vi "Read.vi"(6 "Append Index":i32, 8 "error in (no error)":errorcluster, 11 "DAT in":refnum<class "LV-Data.DAT.lvclass">) -> (0 "error out":errorcluster, 1 "Notes":string, 2 "Data (Dictionary)":T1[](array[typedef]), 3 "DAT out":refnum<class "LV-Data.DAT.lvclass">, 5 "Path out":path)   [LabVIEW 2016, in "LV-Data.DAT.lvclass"]
uses:
  LV-Data.DAT.lvclass
  C:/Users/patrick/Documents/GitHub/LV-to-ITX/src/Data/LV-Data.lvclass
  LV-Data/Typedefs/Dictionary--cluster.ctl
  LV-Data/LV-Data.lvclass/LV-Data.ctl
  <vilib>/Utility/file.llb/Read Delimited Spreadsheet (string).vi
  LV-Data/LV-Data.lvclass
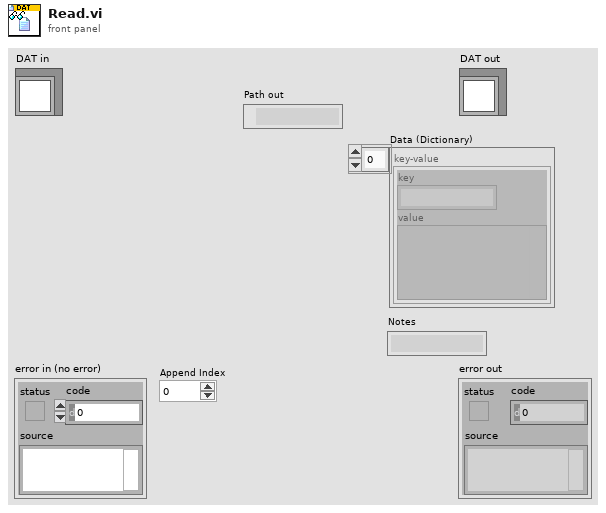
[diagram p1: front panel]
types:
  T1 = typedef "LV-Data.lvclass/Dictionary--cluster.ctl" = cluster{"key":string, "value":variant}
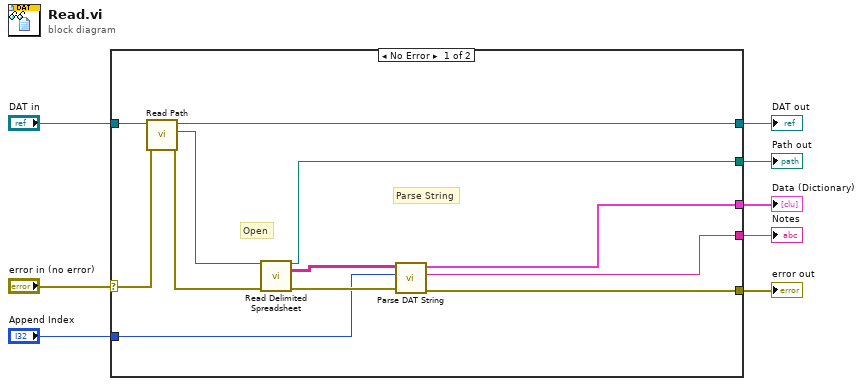
[diagram p0: block diagram]
diagram:
  n1 = case shown="No Error" "error in (no error)" {
    selector: "error in (no error)" -> [w13 w22]
    tunnel: "DAT in" -> [w14 w21]
    tunnel: [w18 w21] -> w7
    tunnel: [w17 w22] -> w6
    tunnel: [w12 _] -> w4
    tunnel: [w11 _] -> w3
    tunnel: [w10 _] -> w2
    tunnel: "Append Index" -> [w9 _]
    frame No Error {
      # "Parse String"
      # "Open"
      n2 = call "Read Path.vi"("error in (no error)"=w13, "Data Save"=w14) -> ("error out"=w19:errorcluster, "Path"=w16:path, "Data Save out"=w18:refnum<class "LV-Data.DAT.lvclass">)  [unwired: 7 in]
      n3 = call-poly <vilib>:"Read Delimited Spreadsheet.vi"("file path (dialog if empty)"=w16, "error in (no error)"=w19) -> ("new file path (Not A Path if cancelled)"=w12:path, "all rows"=w15:string[][], "error out"=w20:errorcluster)  [unwired: 8 in, 3 out]
      n4 = call "Parse DAT String.vi"("error in (no error)"=w20, "header length"=w9, "spreadsheet string"=w15) -> ("error out"=w17:errorcluster, "Notes"=w10:string, "Data (Dictionary)"=w11:T1[])  [unwired: 6 in]
    }
    frame Error {
    }
  }
  "error out" <- w6
  "DAT out" <- w7
  "Path out" <- w4
  "Data (Dictionary)" <- w3
  "Notes" <- w2
